vi "BuscarValores 1columna numerico (SubVI).vi"(0 "Columna?":string="IMEI", 1 "Tabla":string="Tabla1", 2 "Columna":string="POC", 3 "=":string="1") -> (7 "String":string)   [LabVIEW 2012]
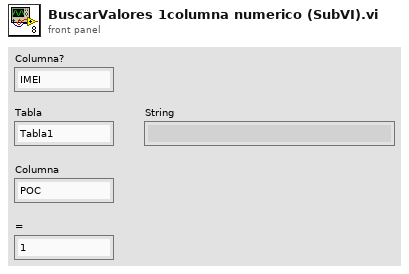
[diagram p1: front panel]
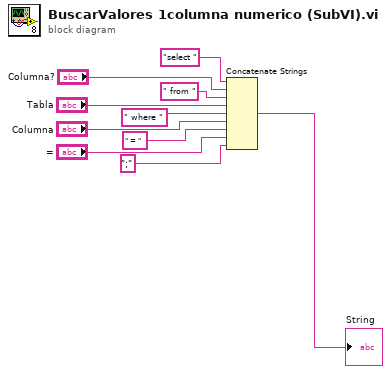
[diagram p0: block diagram]
diagram:
  n1 = Concatenate Strings("select " ("SQL query"), "Columna?", " from " ("SQL query"), "Tabla", " where " ("string"), "Columna", " = " ("Substring"), "=", ";") -> (→"String":string)
